vi "test_Scripting API Messages_Created Message Group.vi"(8 "error in (no error)":errorcluster, 11 "TestCase in":refnum<class "Instrument Addon Scripting API Messages Unit Tests.lvclass">) -> (0 "error out":errorcluster, 3 "TestCase out":refnum<class "Instrument Addon Scripting API Messages Unit Tests.lvclass">)   [LabVIEW 2018, in "Instrument Addon Scripting API Messages Unit Tests.lvclass"]
uses:
  Instrument Addon Scripting API Messages Unit Tests.lvclass
  NationalInstruments.VeriStand.SystemDefinitionAPI
  Addon/Addon Shared/SubVIs/Constants.vi
  <vilib>/addons/_JKI Toolkits/VI Tester/TestCase.llb/TestCase.lvclass
  APIs/Scripting API/Instrument Addon Scripting API.lvlib
  Addon/Addon Shared/Instrument Addon Shared.lvlib
  <vilib>/NI VeriStand/Custom Device API/Custom Device API.lvlib
  C:/Program Files (x86)/National Instruments/LabVIEW 2018/vi.lib/addons/_JKI Toolkits/VI Tester/TestCase.llb/TestCase.lvclass
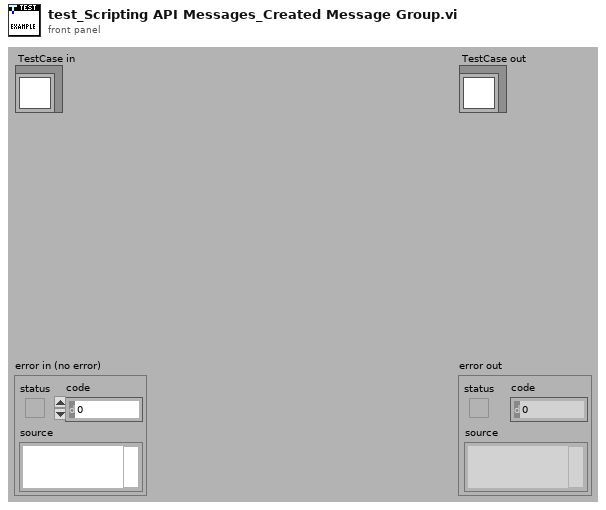
[diagram p1: front panel]
types:
  T1 = typedef "Instrument Addon Refnum In.ctl" = u64
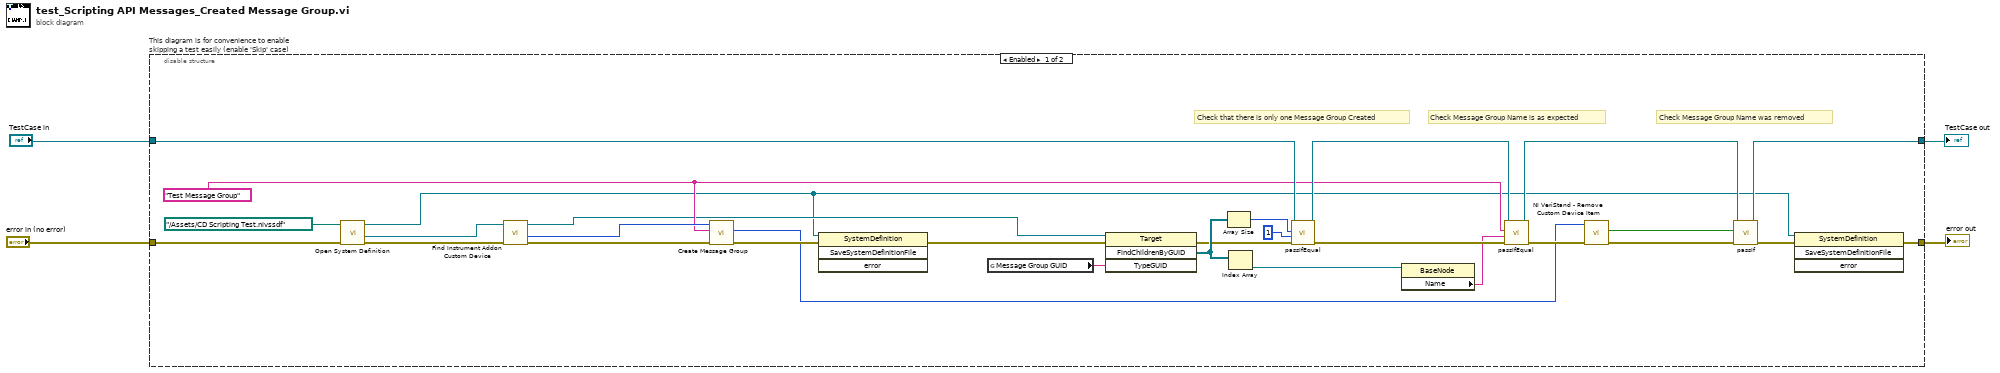
[diagram p0: block diagram]
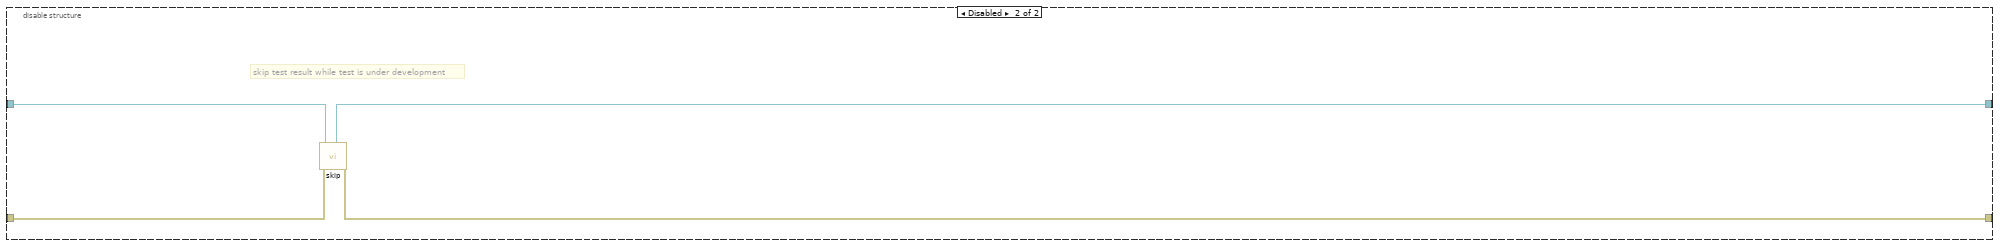
[diagram p2: hidden frame]
diagram:
  n1 = disable-structure "This diagram is for convenience to enable skipping a test easily (enable 'Skip' case)" shown="Enabled" {
    disable-tunnel: "TestCase in" -> [w23 w37]
    disable-tunnel: [w13 w35] -> w1
    disable-tunnel: [w19 w36] -> w3
    disable-tunnel: "error in (no error)" -> [w33 w34]
    frame Enabled {
      w10 = "Test Message Group" ("Section Name")
      # "Check Message Group Name was removed"
      # "Check Message Group Name is as expected"
      # "Check that there is only one Message Group Created"
      n2 = call "Open System Definition.vi"("error in (no error)"=w33, "System Definition File"=path "../Assets/CD Scripting Test.nivssdf" ("SDF file")) -> ("error out"=w31:errorcluster, "Target Refnum"=w32:refnum<k24>, "System Definition Refnum"=w5:refnum<k24>)  [unwired: 6 in, 1 out]
      n3 = call "Find Instrument Addon Custom Device.vi"("error in"=w31, "target in"=w32) -> ("error out"=w11:errorcluster, "NodeID"=w12:u64, "target out"=w7:refnum<k24>)  [unwired: 7 in]
      n4 = call "Create Message Group.vi"("error in (no error)"=w11, "Message Group Name"=w10, "Instrument Addon Refnum In"=w12) -> ("error out"=w9:errorcluster, "Message Group Refnum"=w6:T1)  [unwired: 6 in, 1 out]
      n5 = invoke class="SystemDefinition" method="SaveSystemDefinitionFile"(reference=w5, error in=w9) -> (error out=w8:errorcluster)  [unwired: 2 in, 3 out]
      n6 = global read "Constants.vi" "Message Group GUID"() -> (w29:string)
      n7 = invoke class="Target" method="FindChildrenByGUID"(reference=w7, error in=w8, "TypeGUID"=w29) -> (error out=w25:errorcluster, "FindChildrenByGUID"=w28:refnum<k24>[])  [unwired: 1 in, 2 out]
      n8 = Array Size(array=w28) -> (size(s)=w27:i32)
      n9 = Index Array(array=w28) -> (element=w20:refnum<k24>)  [unwired: 1 in]
      n10 = call-dynamic "passIfEqual.vi"("error in (no error)"=w25, "y"=1 ("size(s)"), "x"=w27, "TestCase in"=w23) -> ("error out"=w24:errorcluster, "TestCase out"=w22:refnum<class "Instrument Addon Scripting API Messages Unit Tests.lvclass">)  [unwired: 6 in]
      n11 = property class="BaseNode"(reference=w20) -> ("Name"=w21:string)  [unwired: 1 in, 2 out]
      n12 = call-dynamic "passIfEqual.vi"("error in (no error)"=w24, "y"=w21, "x"=w10, "TestCase in"=w22) -> ("error out"=w18:errorcluster, "TestCase out"=w14:refnum<class "Instrument Addon Scripting API Messages Unit Tests.lvclass">)  [unwired: 6 in]
      n13 = call <vilib>:"NI VeriStand - Remove Custom Device Item.vi"("error in (no error)"=w18, "Item Ref in"=w6) -> ("error out"=w17:errorcluster, "Deleted?"=w15:bool)  [unwired: 8 in]
      n14 = call-dynamic "passIf.vi"("error in (no error)"=w17, "pass"=w15, "TestCase in"=w14) -> ("error out"=w16:errorcluster, "TestCase out"=w13:refnum<class "Instrument Addon Scripting API Messages Unit Tests.lvclass">)  [unwired: 7 in]
      n15 = invoke class="SystemDefinition" method="SaveSystemDefinitionFile"(reference=w5, error in=w16) -> (error out=w19:errorcluster)  [unwired: 2 in, 3 out]
    }
    frame Disabled {
      # "skip test result while test is under development"
      n16 = call <vilib>:"skip.vi"("error in (no error)"=w34, "TestCase in"=w37) -> ("error out"=w36:errorcluster, "TestCase out"=w35:refnum<class "Instrument Addon Scripting API Messages Unit Tests.lvclass">)  [unwired: 8 in]
    }
  }
  "error out" <- w3
  "TestCase out" <- w1
